vi "事件结构.vi"() -> ()   [LabVIEW 2017]
panel:
  in  "取相反数":bool
  in  "平方根":bool
  in  "除":bool
  in  "乘":bool
  in  "减":bool
  in  "加":bool
  in  "停止":bool
  out "波形图表":dbl(graph)
  in  "数值 4":dbl
  in  "数值 3":dbl
  in  "数值 2":dbl
  in  "数值":dbl
  # "平方根、取相反数"
  # "加减乘除运算"
  # "加、减、乘、除"
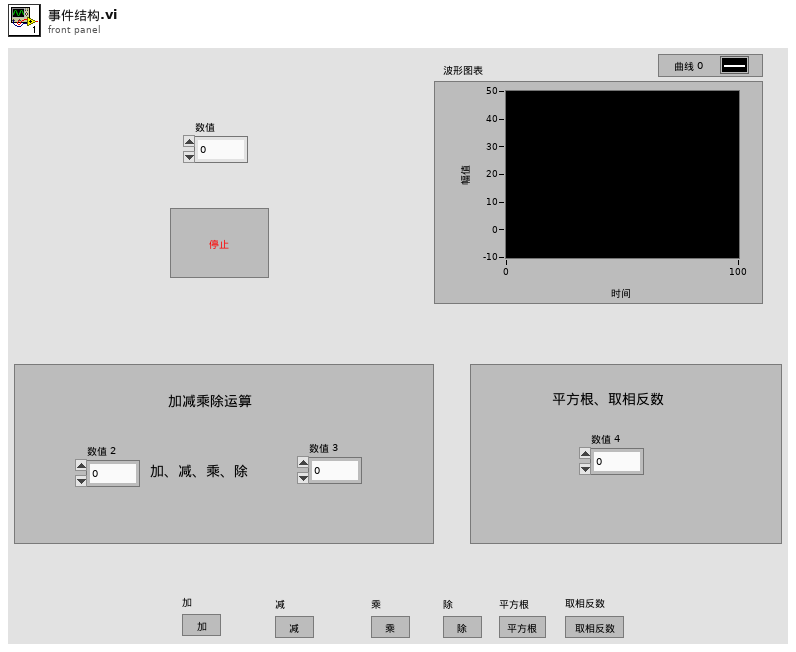
[diagram p1: front panel]
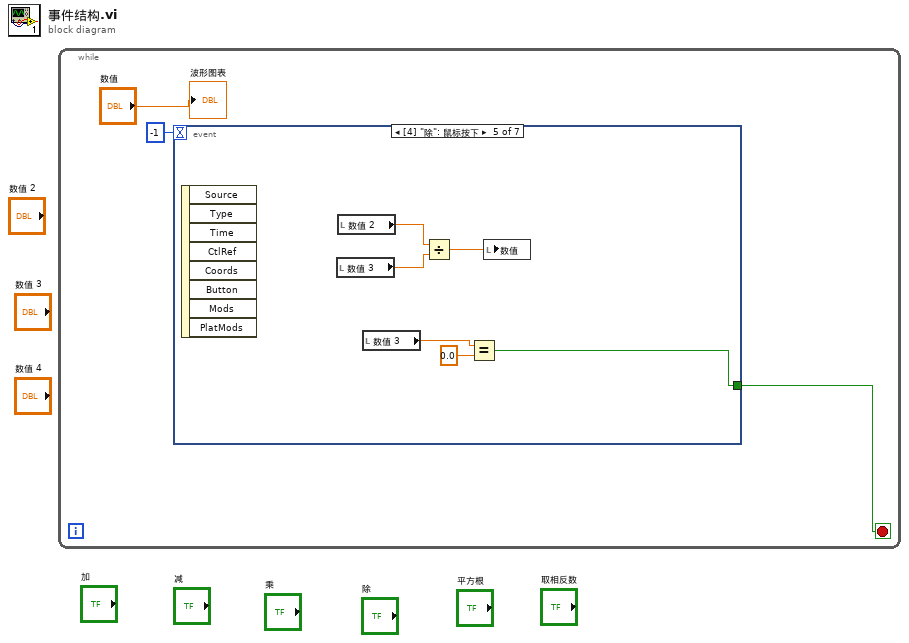
[diagram p0: block diagram]
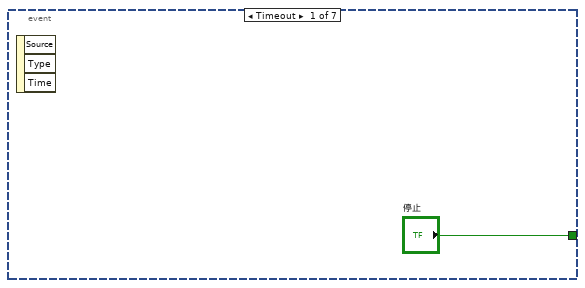
[diagram p2: hidden frame]
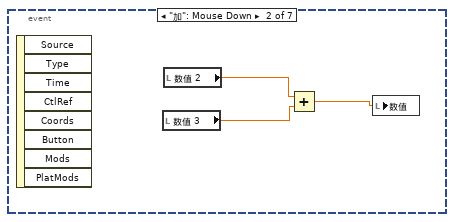
[diagram p3: hidden frame]
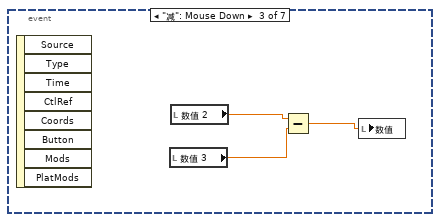
[diagram p4: hidden frame]
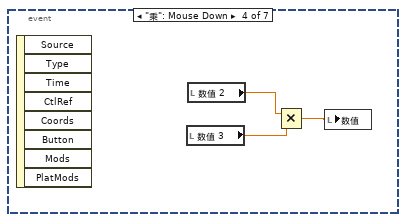
[diagram p5: hidden frame]
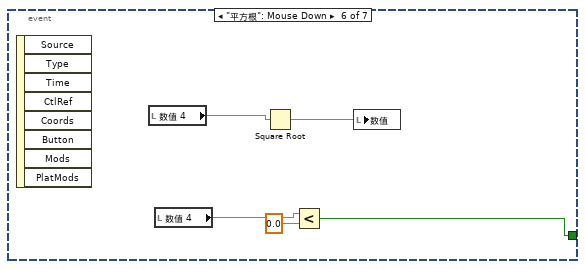
[diagram p6: hidden frame]
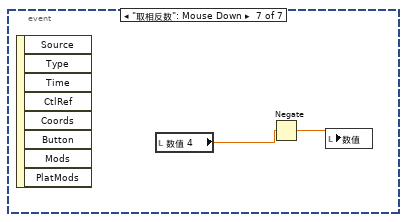
[diagram p7: hidden frame]
diagram:
  n1 = while {
    stop <- w3 stop-if-true
    n2 = event shown="[4] \"除\": 鼠标按下" {
      selector: _ -> [_ _ _ _ _ _ _]
      dyn-events: _ -> [_ _ _ _ _ _ _]
      timeout: -1 -> [_ _ _ _ _ _ _]
      tunnel: ["停止" _ _ _ w14 w20 _] -> w3
      event Timeout {
        n3 = event-data() -> ()  [unwired: 1 in, 3 out]
      }
      event "加": Mouse Down {
        n4 = event-data() -> ()  [unwired: 1 in, 8 out]
        n5 = local read "数值 3"() -> (w6:dbl)
        n6 = local read "数值 2"() -> (w7:dbl)
        n7 = Add(x=w7, y=w6) -> (x+y=w5:dbl)
        n8 = local write "数值"(w5) -> ()
      }
      event "减": Mouse Down {
        n9 = event-data() -> ()  [unwired: 1 in, 8 out]
        n10 = local read "数值 3"() -> (w9:dbl)
        n11 = local read "数值 2"() -> (w10:dbl)
        n12 = Subtract(x=w10, y=w9) -> (x-y=w8:dbl)
        n13 = local write "数值"(w8) -> ()
      }
      event "乘": Mouse Down {
        n14 = event-data() -> ()  [unwired: 1 in, 8 out]
        n15 = local read "数值 3"() -> (w12:dbl)
        n16 = local read "数值 2"() -> (w13:dbl)
        n17 = Multiply(x=w13, y=w12) -> (x*y=w11:dbl)
        n18 = local write "数值"(w11) -> ()
      }
      event "除": Mouse Down {
        n19 = event-data() -> ()  [unwired: 1 in, 8 out]
        n20 = local read "数值 3"() -> (w18:dbl)
        n21 = local read "数值 2"() -> (w19:dbl)
        n22 = local read "数值 3"() -> (w16:dbl)
        n23 = Divide(x=w19, y=w18) -> (x/y=w17:dbl)
        n24 = Equal?(x=w16, y=0.0) -> (x = y?=w14:bool)
        n25 = local write "数值"(w17) -> ()
      }
      event "平方根": Mouse Down {
        n26 = event-data() -> ()  [unwired: 1 in, 8 out]
        n27 = local read "数值 4"() -> (w24:dbl)
        n28 = local read "数值 4"() -> (w22:dbl)
        n29 = Square Root(x=w24) -> (sqrt(x)=w23:dbl)
        n30 = Less?(x=w22, y=0.0) -> (x < y?=w20:bool)
        n31 = local write "数值"(w23) -> ()
      }
      event "取相反数": Mouse Down {
        n32 = event-data() -> ()  [unwired: 1 in, 8 out]
        n33 = local read "数值 4"() -> (w26:dbl)
        n34 = Negate(x=w26) -> (-x=w25:dbl)
        n35 = local write "数值"(w25) -> ()
      }
    }
    "波形图表" <- "数值"
  }
